vi "Calibration.vi"(8 "Error In":errorcluster) -> (0 "Error Out":errorcluster, 3 "Calibration Path Out":path)   [LabVIEW 2017]
doc: "This VI allows the user to calibrate an image for lens distortion, real world dimentions and home the X/Y and Theta Axis."
uses:
  calibration_states.llb/Calibration States.ctl
panel:
  in  "File Path Control":path
  in  "No Calibration":bool
  in  "Open Existing":bool
  in  "New Calibration":bool
  # "Welcome - Group 6"
  # "New Calibration - Take photo and calibrate. Home Axis.\nNo Calibration - Continue without calibration.\nOpen Existing - Open a previously created image calibration file"
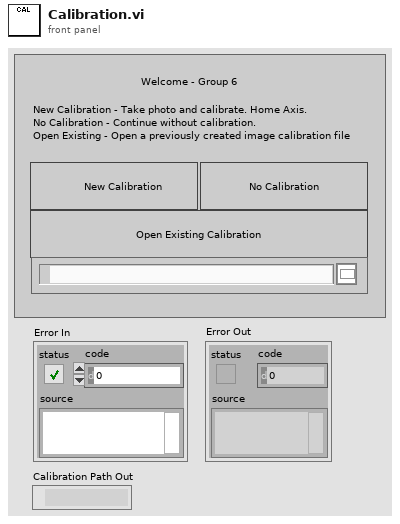
[diagram p1: front panel]
types:
  T1 = typedef "Calibration States.ctl" = cluster{enum16{"Idle", "New", "Open (file)", "Open (no file)", "Close"}, "Message Data":variant}
  T2 = enum16{"Idle", "New", "Open (file)", "Open (no file)", "Close"}
  T3 = cluster{enum16{"Idle", "New", "Open (file)", "Open (no file)", "Close"}, "Variant":variant}
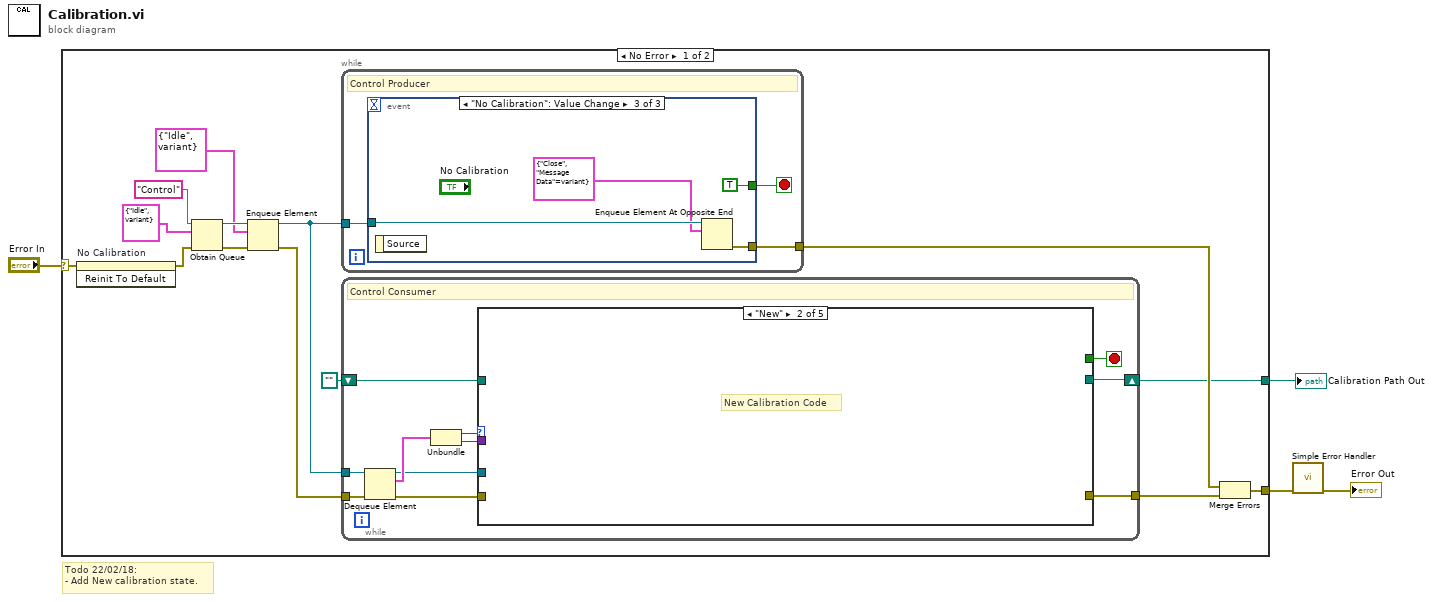
[diagram p0: block diagram]
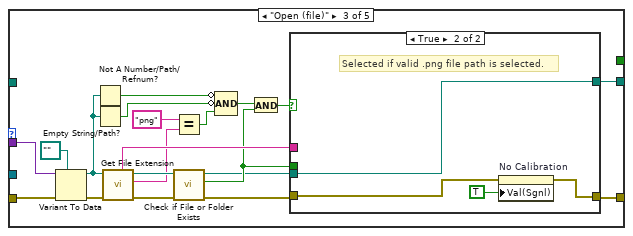
[diagram p3: hidden frame]
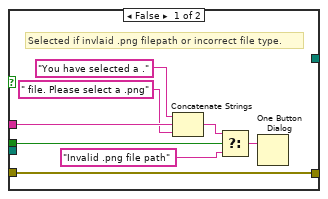
[diagram p4: hidden frame]
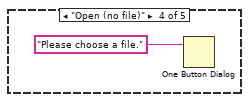
[diagram p5: hidden frame]
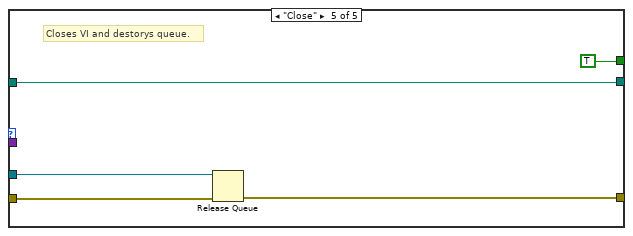
[diagram p6: hidden frame]
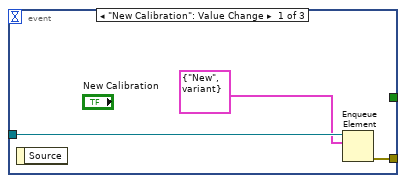
[diagram p7: hidden frame]
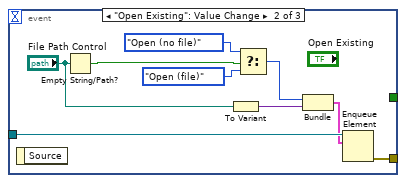
[diagram p8: hidden frame]
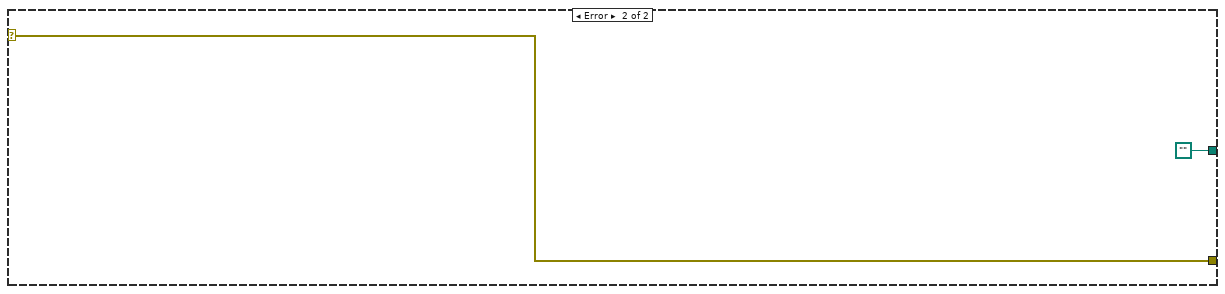
[diagram p9: hidden frame]
diagram:
  # "Todo 22/02/18: \n- Add New calibration state."
  n1 = case shown="No Error" "Error In" {
    selector: "Error In" -> [w8 w88]
    tunnel: [w18 w88] -> w4
    tunnel: [w5 path ""] -> w1
    frame No Error {
      n2 = invoke on="No Calibration" class="Bool (strict)" method="Reinit To Default"(error in=w8) -> (error out=w9:errorcluster)  [unwired: 2 in, 2 out]
      n3 = Obtain Queue(name (unnamed)="Control", element data type=T1 {enum."Idle", "Message Data"=variant}, error in (no error)=w9) -> (queue out=w16:refnum<queue>, error out=w15:errorcluster)  [unwired: 2 in, 1 out]
      n4 = Enqueue Element(queue=w16, element=T1 {enum."Idle", "Message Data"=variant}, error in (no error)=w15) -> (queue out=w12:refnum<queue>, error out=w17:errorcluster)  [unwired: 1 in, 1 out]
      n5 = while {
        tunnel: [w69] -> w14
        tunnel: w12 -> [w68]
        stop <- w70 stop-if-true
        # "Control Producer"
        n6 = event shown="[2] \"No Calibration\": Value Change" {
          selector: _ -> [_ _ _]
          dyn-events: _ -> [_ _ _]
          timeout: _ -> [_ _ _]
          tunnel: [_ _ TRUE] -> w70
          tunnel: w68 -> [w73 w82 w86]
          tunnel: [w72 w81 w85] -> w69
          event "New Calibration": Value Change {
            # "Enqueue an \"Action 1\" message."
            n7 = event-data() -> ()  [unwired: 1 in, 1 out]
            n8 = Enqueue Element(queue=w73, element=T1 {enum."New", "Message Data"=variant}) -> (error out=w72:errorcluster)  [unwired: 2 in, 2 out]
          }
          event "Open Existing": Value Change {
            # "Enqueue an \"Action 2\" message."
            n9 = event-data() -> ()  [unwired: 1 in, 1 out]
            n10 = Empty String/Path?(string/path="File Path Control") -> (empty?=w75:bool)
            n11 = To Variant(anything="File Path Control") -> (Variant=w76:variant)
            n12 = Select(t=T2."Open (no file)", s=w75, f=T2."Open (file)") -> (s? t:f=w80:T2)
            n13 = Bundle(w80, "Variant"=w76) -> (w77:T3)  [unwired: 1 in]
            n14 = Enqueue Element(queue=w82, element=w77) -> (error out=w81:errorcluster)  [unwired: 2 in, 2 out]
          }
          event "No Calibration": Value Change {
            # "Enqueue an \"Exit\" message. Note that the Enqueue Element At Opposite End function is used to place this priority \"Exit\" message at the front of the queue ahead of all other messages."
            n15 = event-data() -> ()  [unwired: 1 in, 1 out]
            n16 = Enqueue Element At Opposite End(queue=w86, element=T1 {enum."Close", "Message Data"=variant}) -> (error out=w85:errorcluster)  [unwired: 2 in, 2 out]
          }
        }
      }
      n17 = while {
        tunnel: w17 -> [w29]
        tunnel: w12 -> [w28]
        tunnel: [w23] -> w10
        shift-right: [w19] -> w5
        shift-left: path "" -> [w20]
        stop <- w22 stop-if-true
        # "Control Consumer"
        n18 = Dequeue Element(queue=w28, error in (no error)=w29) -> (queue out=w24:refnum<queue>, element=w26:T1, error out=w27:errorcluster)  [unwired: 1 in, 1 out]
        n19 = Unbundle(w26) -> (w25:T2, "Message Data"=w21:variant)
        n20 = case shown="\"New\"" w25 {
          tunnel: w27 -> [_ _ w47 _ w67]
          tunnel: w24 -> [_ _ _ _ w64]
          tunnel: [_ _ w43 _ w66] -> w23
          tunnel: [_ _ _ _ TRUE] -> w22
          tunnel: w21 -> [_ _ w48 _ _]
          tunnel: w20 -> [_ _ _ _ w63]
          tunnel: [_ _ w30 _ w63] -> w19
          frame "Idle", Default {
          }
          frame "New" {
            # "New Calibration Code"
          }
          frame "Open (file)" {
            n21 = Variant To Data(error in=w47, type=path "", Variant=w48) -> (data=w40:path, error out=w45:errorcluster)
            n22 = Not A Number/Path/Refnum?(number/path/refnum=w40) -> (NaN/Path/Refnum?=w41:bool)
            n23 = Empty String/Path?(string/path=w40) -> (empty?=w42:bool)
            n24 = call <vilib>:"Get File Extension.vi"("error in (no error)"=w45, "file"=w40) -> ("error out"=w38:errorcluster, "lowercase file extension"=w32:string, "dup file"=w39:path, "unmodified file extension"=w44:string)  [unwired: 5 in, 1 out]
            n25 = Equal?(x="png" ("y"), y=w32) -> (x = y?=w49:bool)
            n26 = call <vilib>:"Check if File or Folder Exists.vi"("error in (no error)"=w38, "path"=w39) -> ("error out"=w37:errorcluster, "file or folder exists?"=w34:bool, "dup path"=w31:path)  [unwired: 7 in]
            n27 = Compound Arithmetic op=AND(invert w41, invert w42, w49) -> (w36:bool)
            n28 = And(x=w36, y=w34) -> (x .and. y?=w35:bool)
            n29 = case shown="True" w35 {
              tunnel: w44 -> [w57 _]
              tunnel: w37 -> [w54 w60]
              tunnel: [w54 w59] -> w43
              tunnel: w34 -> [w51 _]
              tunnel: w31 -> [_ w58]
              tunnel: [_ w58] -> w30
              frame False {
                # "Selected if invlaid .png filepath or incorrect file type."
                n30 = Concatenate Strings("You have selected a ." ("message"), w57, " file. Please select a .png" ("string")) -> (w52:string)
                n31 = Select(t=w52, s=w51, f="Invalid .png file path" ("string")) -> (s? t:f=w50:string)
                n32 = One Button Dialog(message=w50) -> ()  [unwired: 1 in, 1 out]
              }
              frame True {
                # "Selected if valid .png file path is selected."
                n33 = property on="No Calibration" class="Bool (strict)"(error in=w60, "Val(Sgnl)"=TRUE ("No Calibration")) -> (error out=w59:errorcluster)  [unwired: 1 in, 1 out]
              }
            }
          }
          frame "Open (no file)" {
            n34 = One Button Dialog(message="Please choose a file.") -> ()  [unwired: 1 in, 1 out]
          }
          frame "Close" {
            # "Closes VI and destorys queue."
            n35 = Release Queue(queue=w64, error in (no error)=w67) -> (error out=w66:errorcluster)  [unwired: 1 in, 2 out]
          }
        }
      }
      n36 = Merge Errors(w14, w10) -> (w18:errorcluster)
    }
    frame Error {
    }
  }
  "Calibration Path Out" <- w1
  n37 = call <vilib>:"Simple Error Handler.vi"("error in (no error)"=w4) -> ("error out"=→"Error Out":errorcluster)  [unwired: 4 in, 4 out]
